vi "GetClusterValue.vi"(0 "VI Reference":refnum<vi>, 7 "Array":string[](array[string]), 11 "error in":errorcluster) -> (4 "VI Reference out":refnum<vi>, 8 "Value":variant, 15 "error out":errorcluster)   [LabVIEW 2016]
doc: "This VI gets the specified controls value from other VI. Highly used for Cluster and tab"
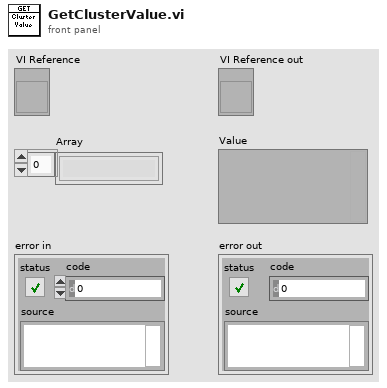
[diagram p1: front panel]
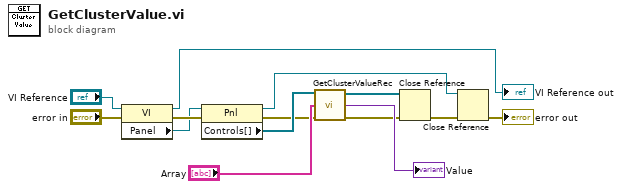
[diagram p0: block diagram]
diagram:
  n1 = property class="VI"(reference="VI Reference", error in="error in") -> (reference out=→"VI Reference out":refnum<vi>, error out=w14:errorcluster, "Panel"=w13:refnum<vi>)
  n2 = property class="Pnl"(reference=w13, error in=w14) -> (reference out=w8:refnum<vi>, error out=w3:errorcluster, "Controls[]"=w6:refnum<vi>[])
  n3 = call "GetClusterValueRec.vi"("Controls[] In"=w6, "Array"="Array", "error in (no error)"=w3) -> ("Controls[] Out"=w1:refnum<vi>[], "Control Value"=→"Value":variant, "error out"=w2:errorcluster)  [unwired: 10 in]
  n4 = Close Reference(reference=w1, error in (no error)=w2) -> (error out=w7:errorcluster)
  n5 = Close Reference(reference=w8, error in (no error)=w7) -> (error out=→"error out":errorcluster)
